vi "test_Find Equation Variables_no values as inputs.vi"(8 "error in (no error)":errorcluster, 11 "TestCase in":refnum<class "Instrument Addon Unit Tests.lvclass">) -> (0 "error out":errorcluster, 3 "TestCase out":refnum<class "Instrument Addon Unit Tests.lvclass">)   [LabVIEW 2020, in "Instrument Addon Unit Tests.lvclass"]
uses:
  Instrument Addon Unit Tests.lvclass
  <vilib>/addons/_JKI Toolkits/VI Tester/TestCase.llb/TestCase.lvclass
  Addon/Addon System Explorer/Instrument Addon System Explorer.lvlib
  C:/Program Files (x86)/National Instruments/LabVIEW 2020/vi.lib/addons/_JKI Toolkits/VI Tester/TestCase.llb/TestCase.lvclass
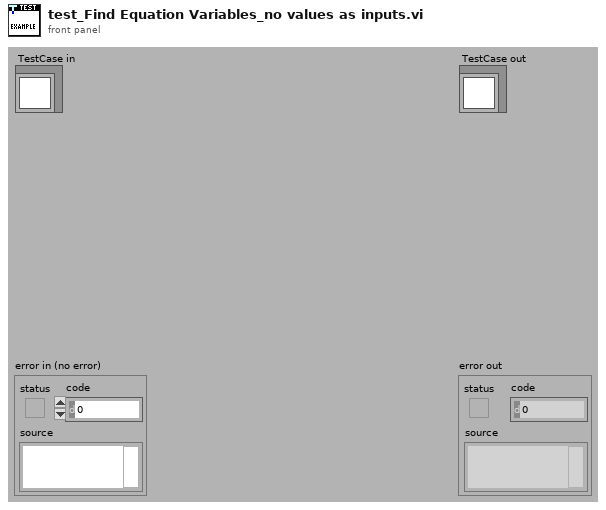
[diagram p1: front panel]
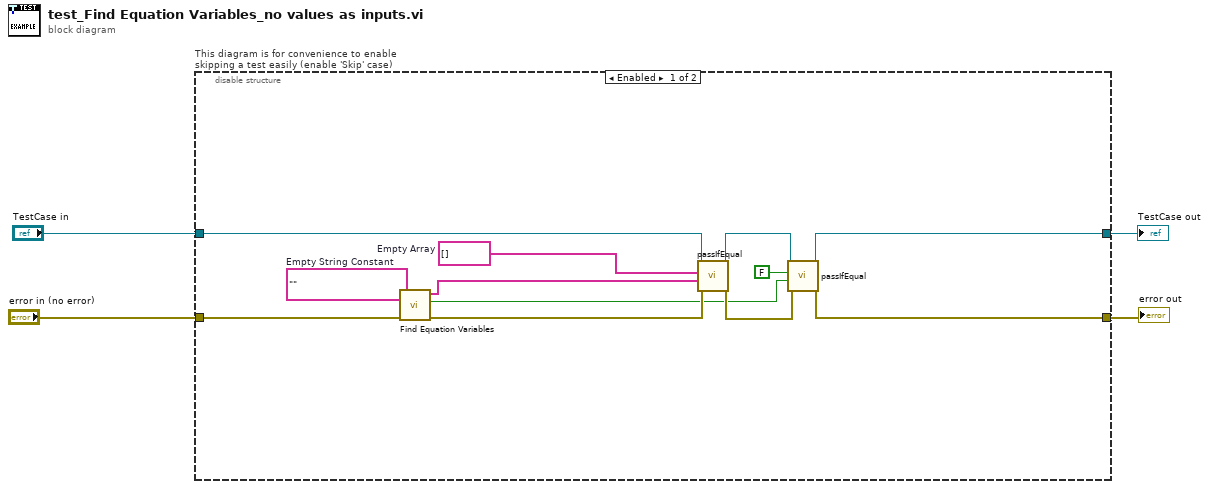
[diagram p0: block diagram]
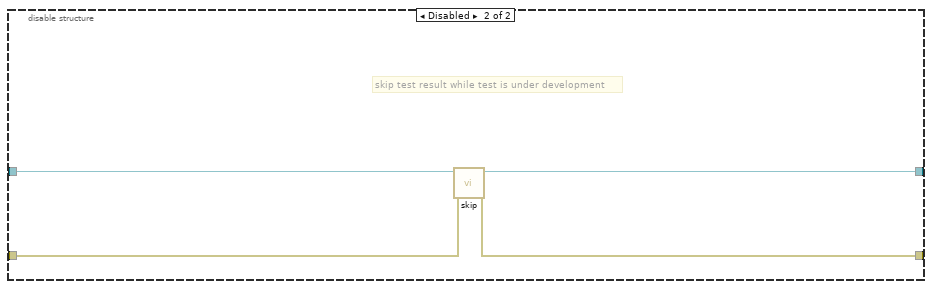
[diagram p2: hidden frame]
diagram:
  n1 = disable-structure "This diagram is for convenience to enable skipping a test easily (enable 'Skip' case)" shown="Enabled" {
    disable-tunnel: "TestCase in" -> [w16 w20]
    disable-tunnel: [w6 w18] -> w1
    disable-tunnel: [w5 w19] -> w3
    disable-tunnel: "error in (no error)" -> [w15 w17]
    frame Enabled {
      w11 = ""  # Empty String Constant
      w12 = string[] []  # Empty Array
      n2 = call "Find Equation Variables.vi"("error in (no error)"=w15, "Command"=w11) -> ("error out"=w14:errorcluster, "Duplicate?"=w9:bool, "Variables"=w13:string[])  [unwired: 7 in]
      n3 = call-dynamic "passIfEqual.vi"("error in (no error)"=w14, "y"=w13, "x"=w12, "TestCase in"=w16) -> ("error out"=w10:errorcluster, "TestCase out"=w7:refnum<class "Instrument Addon Unit Tests.lvclass">)  [unwired: 6 in]
      n4 = call-dynamic "passIfEqual.vi"("error in (no error)"=w10, "y"=w9, "x"=FALSE, "TestCase in"=w7) -> ("error out"=w5:errorcluster, "TestCase out"=w6:refnum<class "Instrument Addon Unit Tests.lvclass">)  [unwired: 6 in]
    }
    frame Disabled {
      # "skip test result while test is under development"
      n5 = call <vilib>:"skip.vi"("error in (no error)"=w17, "TestCase in"=w20) -> ("error out"=w19:errorcluster, "TestCase out"=w18:refnum<class "Instrument Addon Unit Tests.lvclass">)  [unwired: 8 in]
    }
  }
  "error out" <- w3
  "TestCase out" <- w1
